vi "Connect.vi"(8 "error in (no error)":errorcluster, 11 "InferenceTCP in":refnum<class "InferenceTCP.lvclass">) -> (0 "error out":errorcluster, 3 "InferenceTCP out":refnum<class "InferenceTCP.lvclass">)   [LabVIEW 2021, in "InferenceTCP.lvlib" / "InferenceTCP.lvclass"]
uses:
  InferenceTCP.lvclass
  InferenceTCP.lvclass/InferenceTCP.ctl
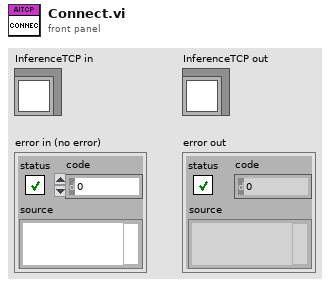
[diagram p1: front panel]
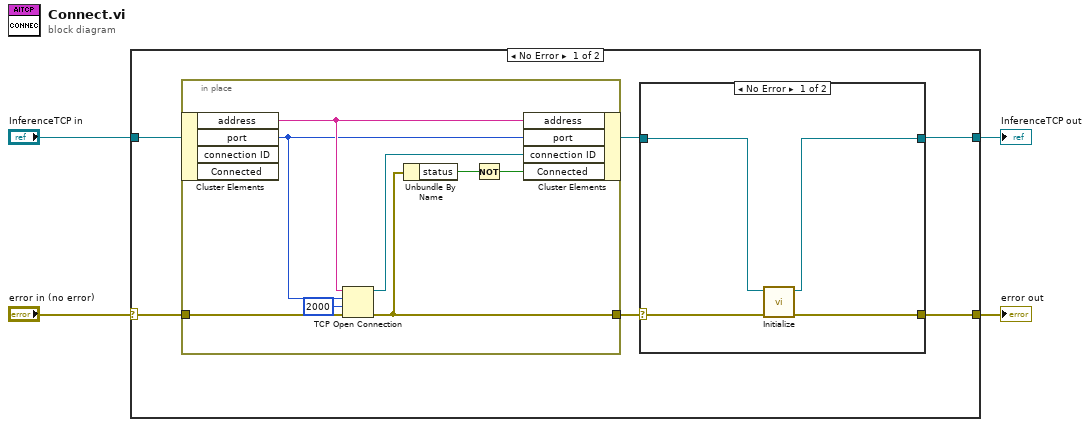
[diagram p0: block diagram]
diagram:
  n1 = case shown="No Error" "error in (no error)" {
    selector: "error in (no error)" -> [w9 w26]
    tunnel: [w5 w26] -> w3
    tunnel: [w6 w25] -> w1
    tunnel: "InferenceTCP in" -> [w10 w25]
    frame No Error {
      n2 = in-place {
        in-place-border: w9 -> [w24]
        in-place-border: [w20] -> w8
        n3 = in-place-cluster #1(w10) -> ("address"=w23:string, "port"=w22:u16)  [unwired: 2 out]
        n4 = TCP Open Connection(address=w23, remote port or service name=w22, timeout ms (60000)=2000, error in (no error)=w24) -> (connection ID=w21:refnum<k5>, error out=w20:errorcluster)  [unwired: 1 in]
        n5 = Unbundle By Name(w20) -> ("status"=w19:bool)
        n6 = Not(x=w19) -> (.not. x?=w18:bool)
        n7 = in-place-cluster #1("address"=w23, "port"=w22, "connection ID"=w21, "Connected"=w18) -> (w7:refnum<class "InferenceTCP.lvclass">)
      }
      n8 = case shown="No Error" w8 {
        selector: w8 -> [w13 w15]
        tunnel: w7 -> [w14 w16]
        tunnel: [w12 w16] -> w6
        tunnel: [w11 w15] -> w5
        frame No Error {
          n9 = call "Initialize.vi"("error in (no error)"=w13, "InferenceTCP in"=w14) -> ("error out"=w11:errorcluster, "InferenceTCP out"=w12:refnum<class "InferenceTCP.lvclass">)  [unwired: 8 in]
        }
        frame Error {
        }
      }
    }
    frame Error {
    }
  }
  "error out" <- w3
  "InferenceTCP out" <- w1
